vi "Drawing Pad.vi"(8 "에러 입력":errorcluster) -> (0 "에러 출력":errorcluster, 3 "이미지 데이터":cluster{"Red":u8, "Green":u8, "Blue":u8}[][](array[cluster]))   [LabVIEW 2018]
uses:
  <vilib>/Utility/cursorutil.llb/Set Cursor (Icon Pict).vi
panel:
  in  "Clear":bool caption="지우기"
  in  "Pen Color":u32(colorbox) caption="펜 색"
  in  "Done":bool caption="완료"
  out "그림":picture
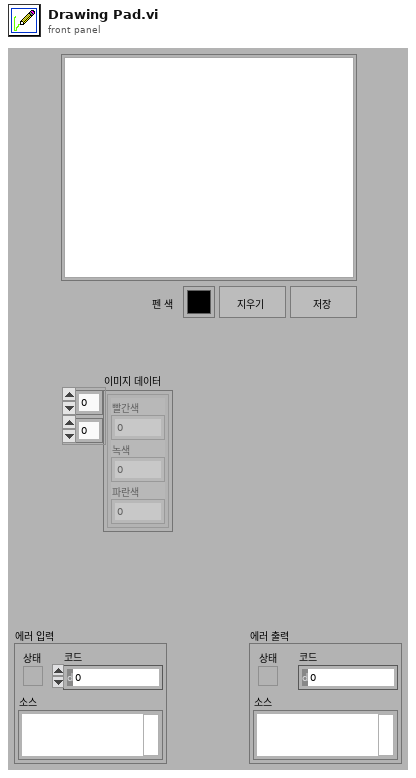
[diagram p1: front panel]
types:
  T1 = typedef "LVPoint32TypeDef.ctl" = cluster{"Horizontal":i32, "Vertical":i32}
  T2 = typedef "LVBoundsTypeDef.ctl" = cluster{"Width":u32, "Height":u32}
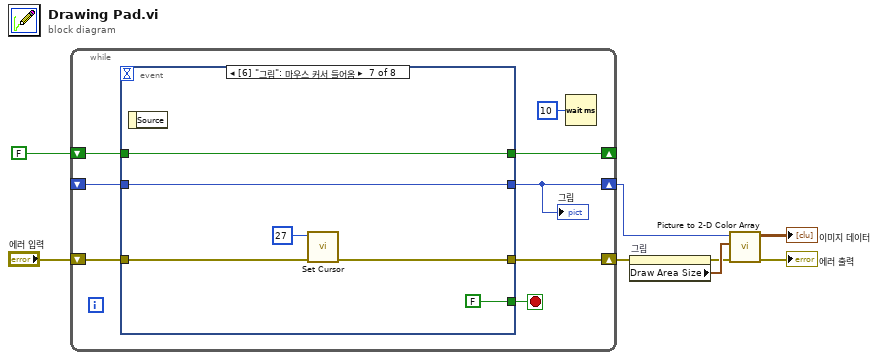
[diagram p0: block diagram]
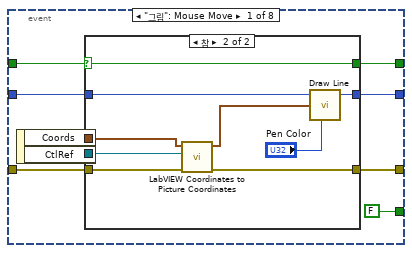
[diagram p2: hidden frame]
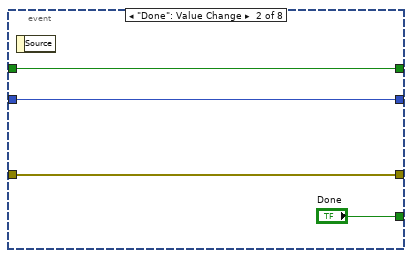
[diagram p4: hidden frame]
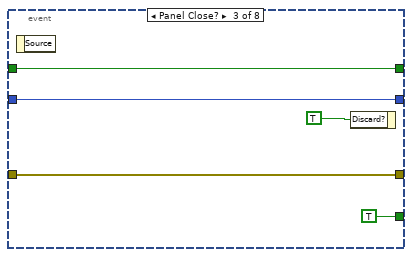
[diagram p5: hidden frame]
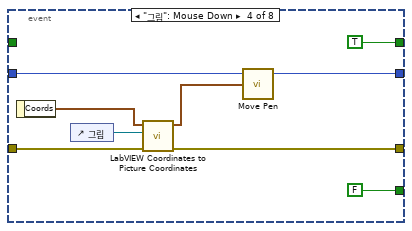
[diagram p6: hidden frame]
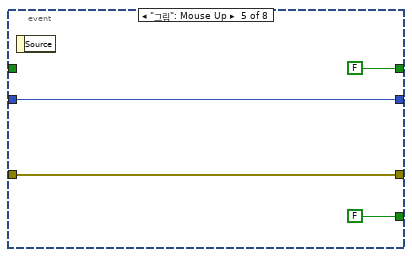
[diagram p7: hidden frame]
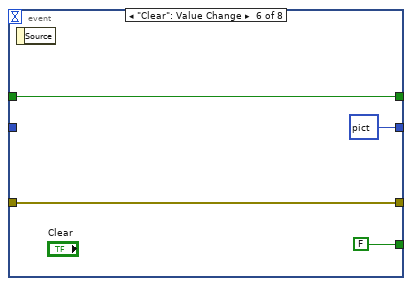
[diagram p8: hidden frame]
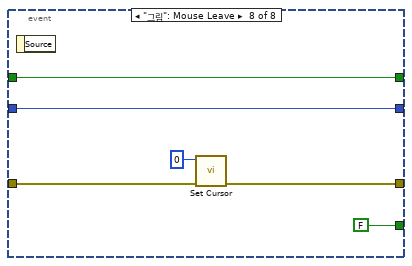
[diagram p9: hidden frame]
diagram:
  n1 = while {
    shift-right: [w14] -> _
    shift-left: FALSE -> [w16]
    shift-right: [w13] -> w2
    shift-left: "에러 입력" -> [w12]
    shift-right: [w10] -> w5
    shift-left: _ -> [w11]
    stop <- w15 stop-if-true
    n2 = event shown="[6] \"그림\": 마우스 커서 들어옴" {
      selector: _ -> [_ _ _ _ _ _ _ _]
      dyn-events: _ -> [_ _ _ _ _ _ _ _]
      timeout: _ -> [_ _ _ _ _ _ _ _]
      tunnel: w16 -> [w25 w40 w46 _ _ w62 w65 w72]
      tunnel: [FALSE ("Done") "Done" TRUE ("Done") FALSE FALSE FALSE ("Done") FALSE ("Done") FALSE ("Done")] -> w15
      tunnel: [w24 w40 w46 TRUE FALSE w62 w65 w72] -> w14
      tunnel: [w18 w38 w44 w48 w56 w61 w68 w74] -> w13
      tunnel: w12 -> [w19 w38 w44 w49 w56 w61 w67 w73]
      tunnel: [w23 w39 w45 w50 w57 picture data[5B] ("new picture") w66 w71] -> w10
      tunnel: w11 -> [w22 w39 w45 w51 w57 _ w66 w71]
      event "그림": Mouse Move {
        n3 = event-data() -> ("Coords"=w21:T1, "CtlRef"=w20:refnum<vi>)  [unwired: 1 in]
        n4 = case shown="참" w25 {
          selector: w25 -> [w28 w37]
          tunnel: [w28 w37] -> w24
          tunnel: [w27 w36] -> w23
          tunnel: w22 -> [w27 w35]
          tunnel: w21 -> [_ w30]
          tunnel: w20 -> [_ w31]
          tunnel: w19 -> [w26 w33]
          tunnel: [w26 w32] -> w18
          frame False {
          }
          frame True {
            n5 = call "LabVIEW Coordinates to Picture Coordinates.vi"("에러 입력"=w33, "컨트롤 참조"=w31, "LabVIEW 좌표계"=w30) -> ("에러 출력"=w32:errorcluster, "그림 컨트롤 좌표계"=w29:cluster{"Horizontal":i32, "Vertical":i32})  [unwired: 7 in]
            n6 = call <vilib>:"Draw Line.vi"("picture"=w35, "end point"=w29, "color(black)"="Pen Color") -> ("new picture"=w36:picture)  [unwired: 6 in]
          }
        }
      }
      event "Done": Value Change {
        n7 = event-data() -> ()  [unwired: 1 in, 1 out]
      }
      event Panel Close? {
        n8 = event-data() -> ()  [unwired: 1 in, 1 out]
        n9 = event-data("Discard?"=TRUE) -> ()  [unwired: 1 in, 1 out]
      }
      event "그림": Mouse Down {
        n10 = event-data() -> ("Coords"=w53:T1)  [unwired: 1 in]
        n11 = control-ref of="그림"() -> (w52:refnum<vi>)
        n12 = call "LabVIEW Coordinates to Picture Coordinates.vi"("에러 입력"=w49, "컨트롤 참조"=w52, "LabVIEW 좌표계"=w53) -> ("에러 출력"=w48:errorcluster, "그림 컨트롤 좌표계"=w47:cluster{"Horizontal":i32, "Vertical":i32})  [unwired: 7 in]
        n13 = call <vilib>:"Move Pen.vi"("new position"=w47, "picture"=w51) -> ("new picture"=w50:picture)  [unwired: 3 in]
      }
      event "그림": Mouse Up {
        n14 = event-data() -> ()  [unwired: 1 in, 1 out]
      }
      event "Clear": Value Change {
        n15 = event-data() -> ()  [unwired: 1 in, 1 out]
      }
      event "그림": Mouse Enter {
        n16 = event-data() -> ()  [unwired: 1 in, 1 out]
        n17 = call-poly <vilib>:"Set Cursor.vi"("error in (no error)"=w67, "icon"=u16 27) -> ("error out"=w68:errorcluster)  [unwired: 8 in, 1 out]
      }
      event "그림": Mouse Leave {
        n18 = event-data() -> ()  [unwired: 1 in, 1 out]
        n19 = call-poly <vilib>:"Set Cursor.vi"("error in (no error)"=w73, "icon"=u16 0) -> ("error out"=w74:errorcluster)  [unwired: 8 in, 1 out]
      }
    }
    "그림" <- w10
    n20 = Wait (ms)(milliseconds to wait=u32 10) -> ()  [unwired: 1 out]
  }
  n21 = property on="그림" class="Pict"(error in=w2) -> (error out=w1:errorcluster, "Draw Area Size"=w3:T2)  [unwired: 1 in, 1 out]
  n22 = call "Picture to 2-D Color Array.vi"("에러 입력"=w1, "입력 클러스터"=w3, "그림"=w5) -> ("에러 출력"=→"에러 출력":errorcluster, "색 배열"=→"이미지 데이터":cluster{"Red":u8, "Green":u8, "Blue":u8}[][])  [unwired: 7 in]
